vi "SM motor repeat TDC DS345 tw 2 soft.vi"(0 "SM Config":T5={"VISA Serial ref"="COM3", "Motor Config"={"DriveRatio (mm/rev)"=10.16, "PosLimit + (mm)"=200.0, "PosLimit - (mm)"=0.0, "EncoderRatio (count/rev)"=2000.0, "MotorType"=enum."SM17"}} {"Motor Config"."EncoderRatio (count/rev)" format="%.2f"; "Motor Config"."PosLimit - (mm)" format="%.3f"; "Motor Config"."PosLimit + (mm)" format="%.3f"; "Motor Config"."DriveRatio (mm/rev)" format="%.2f"}, 1 "Waiting time (s)":dbl=3.0, 2 "Sonication position (mm)":dbl, 3 "Moving times":dbl, 4 "Stop motion":bool, 5 "SM setting":T4={"Acceleration (mm/sec^2)"=1000.0, "Velocity (mm/sec)"=1.0, "Position (mm)"=0.0} {"Position (mm)" format="%.3f"; "Velocity (mm/sec)" format="%.3f"; "Acceleration (mm/sec^2)" format="%.3f"}, 6 "Lasting time (s)":dbl=5.0, 7 "Serial":i32=83858441, 9 "Moving parameters":T2={"Velocity (mm/s)"=0.5, "Abs position (mm)"=0.0, "Lasting time (s)"=25.0}, 11 "SRS DS345 GPIB address":string="0:18", 12 "Default setting (DS345)":T1={"Osc. Amp. (V)"=0.01, "Osc. Freq. (Hz)"=1000.0} {"Osc. Freq. (Hz)" min=0.001 max=250000.0 step=0.001 format="%.3f"; "Osc. Amp. (V)" min=0.0 max=0.1 step=0.001 format="%.3f"}, 13 "Cluster":T1={"Osc. Amp. (V)"=0.06, "Osc. Freq. (Hz)"=1200.0} {"Osc. Freq. (Hz)" min=0.001 max=250000.0 step=0.001 format="%.3f"; "Osc. Amp. (V)" min=0.0 max=10.0 step=0.001 format="%.3f"}, 14 "Move":bool) -> (10 "Status":T3, 15 "Position (mm)":dbl)   [LabVIEW 2015]
uses:
  magnetometers/smi/labview/CPM20Software/SmartMotor.llb/SM Config.ctl
  magnetometers/smi/labview/CPM20Software/SmartMotor.llb/SM MotorConfig.ctl
  magnetometers/smi/labview/CPM20Software/SmartMotor.llb/SM Status.ctl
  Global vab.vi
panel:
  in  "Sonication":bool
  out "Ccurrent times":dbl
  in  "Action":bool
  # "SM motor setting"
  # "TDC001 motor information"
  # "DS345 information"
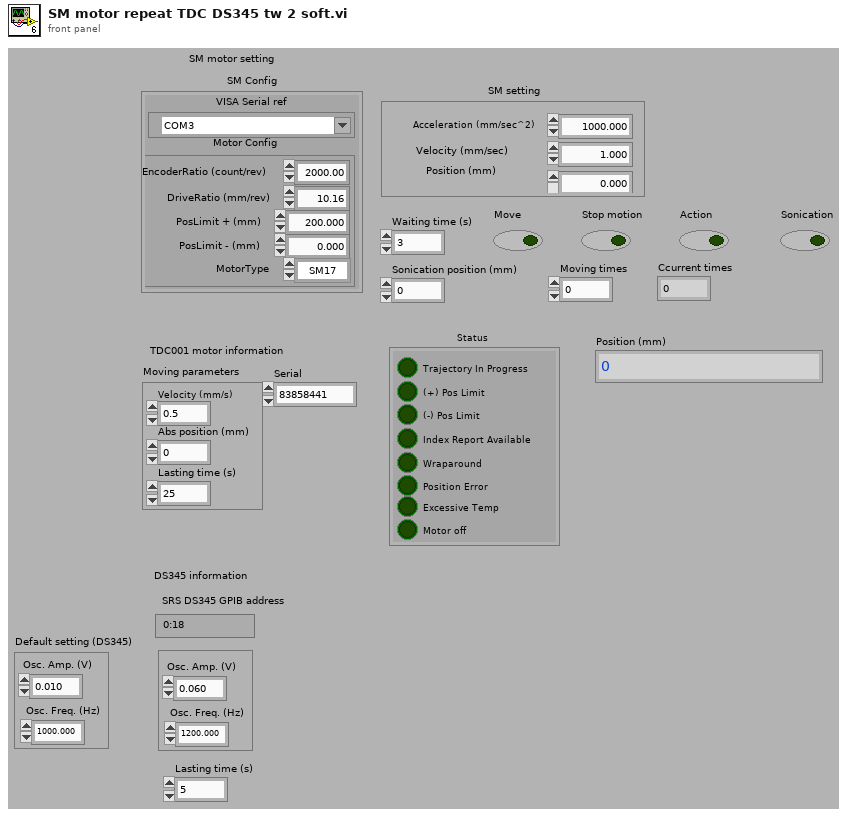
[diagram p1: front panel]
types:
  T1 = cluster{"Osc. Amp. (V)":dbl, "Osc. Freq. (Hz)":dbl}
  T2 = cluster{"Velocity (mm/s)":dbl, "Abs position (mm)":dbl, "Lasting time (s)":dbl}
  T3 = typedef "SM Status.ctl" = cluster{"Trajectory In Progress":bool, "(+) Pos Limit":bool, "(-) Pos Limit":bool, "Index Report Available":bool, "Wraparound":bool, "Position Error":bool, "Excessive Temp":bool, "Motor off":bool}
  T4 = cluster{"Acceleration (mm/sec^2)":dbl, "Velocity (mm/sec)":dbl, "Position (mm)":dbl}
  T5 = typedef "SM Config.ctl" = cluster{"VISA Serial ref":refnum<visa-resource-name>, "Motor Config":T6}
  T6 = typedef "SM MotorConfig.ctl" = cluster{"DriveRatio (mm/rev)":dbl, "PosLimit + (mm)":dbl, "PosLimit - (mm)":dbl, "EncoderRatio (count/rev)":dbl, "MotorType":enum16{"SM17", "SM23", "SM34", "SM42", "SM56"}}
  T7 = cluster{"Acceleration (mm/sec^2)":dbl, "Velocity (mm/sec)":dbl, "Sonication position (mm)":dbl}
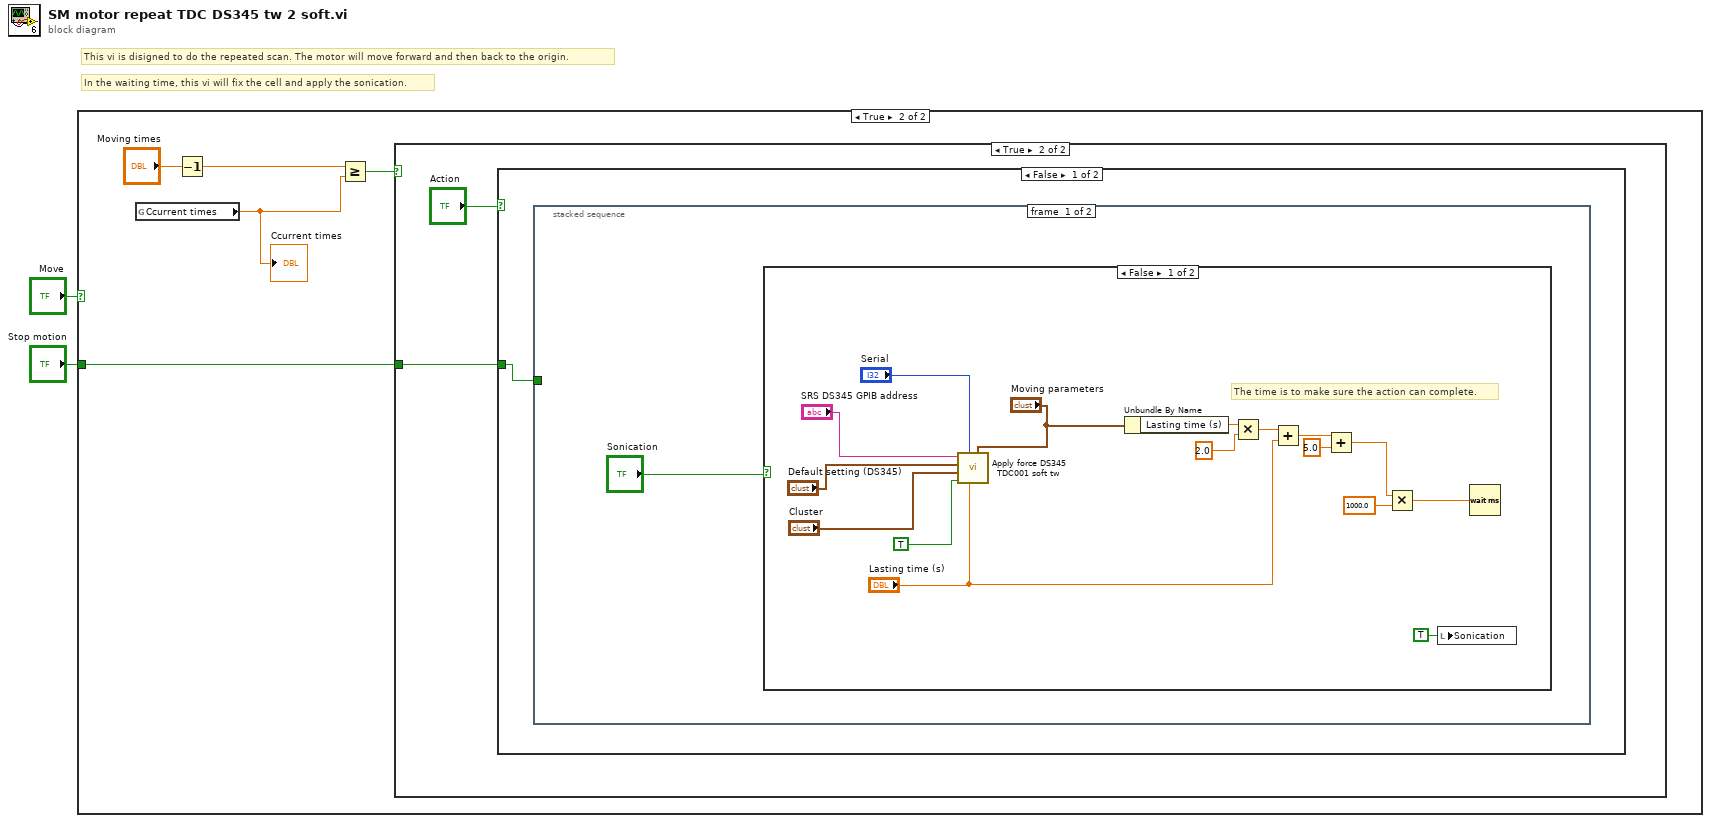
[diagram p0: block diagram]
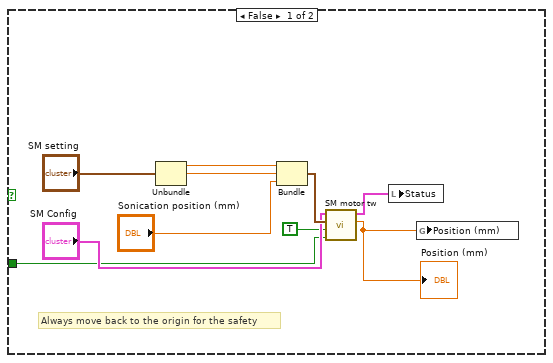
[diagram p2: hidden frame]
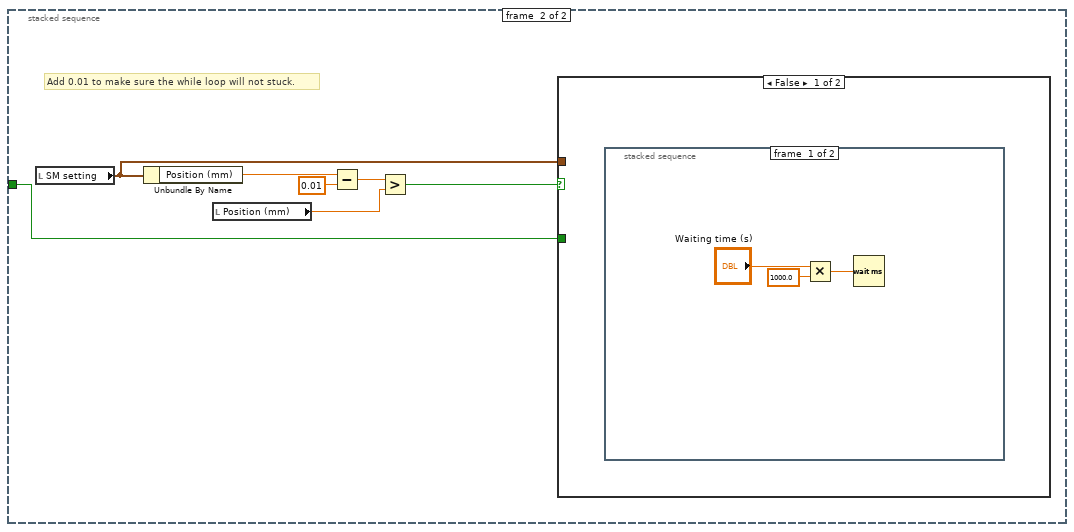
[diagram p5: hidden frame]
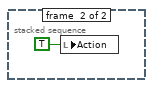
[diagram p6: hidden frame]
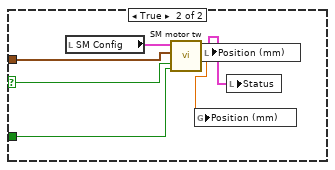
[diagram p7: hidden frame]
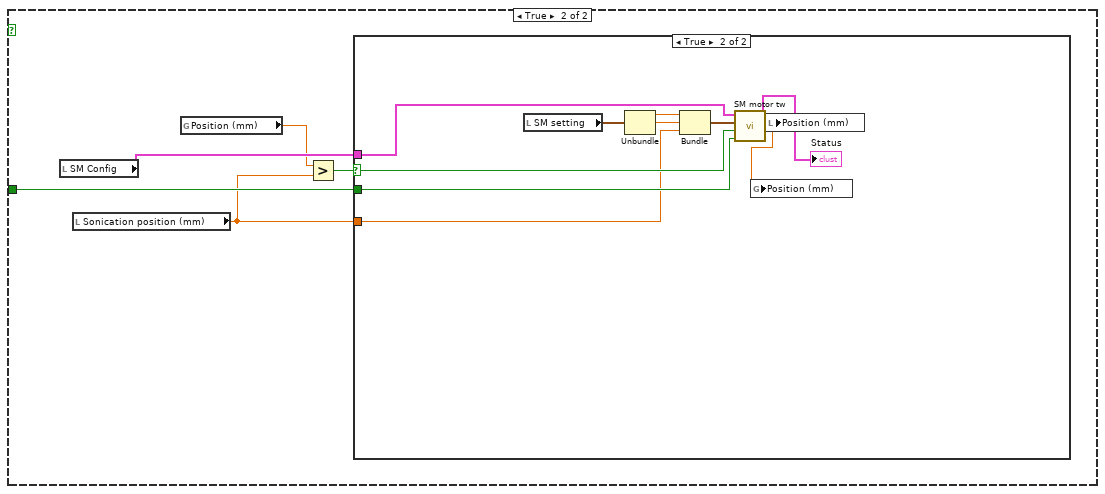
[diagram p8: hidden frame]
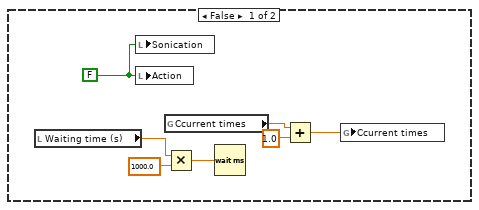
[diagram p9: hidden frame]
diagram:
  # "In the waiting time, this vi will fix the cell and apply the sonication."
  # "This vi is disigned to do the repeated scan. The motor will move forward and then back to the origin."
  n1 = case shown="True" "Move" {
    tunnel: "Stop motion" -> [w6 w15]
    frame False {
      # "Always move back to the origin for the safety"
      n2 = Unbundle("SM setting") -> ("Acceleration (mm/sec^2)"=w12:dbl, "Velocity (mm/sec)"=w11:dbl)  [unwired: 1 out]
      n3 = Bundle("Acceleration (mm/sec^2)"=w12, "Velocity (mm/sec)"=w11, "Sonication position (mm)"="Sonication position (mm)") -> (w10:T7)  [unwired: 1 out]
      n4 = call "SM motor tw.vi"("SM Config"="SM Config", "SM setting"=w10, "Move"=TRUE, "Stop motion"=w6) -> ("Status"=w4:T3, "Position (mm)"=w5:dbl)  [unwired: 5 out]
      "Position (mm)" <- w5
      n5 = local write "Status"(w4) -> ()
      n6 = global write "Global vab.vi" "Position (mm)"(w5) -> ()
    }
    frame True {
      n7 = global read "Global vab.vi" "Ccurrent times"() -> (w13:dbl)
      "Ccurrent times" <- w13
      n8 = Decrement(x="Moving times") -> (x-1=w14:dbl)
      n9 = Greater Or Equal?(x=w14, y=w13) -> (x >= y?=w16:bool)
      n10 = case shown="True" w16 {
        tunnel: w15 -> [_ w19]
        frame False {
        }
        frame True {
          n11 = case shown="False" "Action" {
            tunnel: w19 -> [w20 w57]
            frame False {
              n12 = stacked-sequence {
                tunnel: w20 -> [_ w39]
                frame #0 {
                  n13 = case shown="False" "Sonication" {
                    frame False {
                      # "The time is to make sure the action can complete."
                      n14 = call "Apply force DS345 TDC001 soft tw.vi"("Moving parameters"="Moving parameters", "Lasting time (s)"="Lasting time (s)", "TDC001 motor Serial"="Serial", "Apply force"=TRUE, "Cluster"="Cluster", "Default setting (DS345)"="Default setting (DS345)", "SRS DS345 GPIB address"="SRS DS345 GPIB address") -> ()  [unwired: 4 in]
                      n15 = Unbundle By Name("Moving parameters") -> ("Lasting time (s)"=w28:dbl)
                      n16 = Multiply(x=w28, y=2.0) -> (x*y=w26:dbl)
                      n17 = Add(x=w26, y="Lasting time (s)") -> (x+y=w24:dbl)
                      n18 = Add(x=w24, y=5.0) -> (x+y=w22:dbl)
                      n19 = Multiply(x=w22, y=1000.0) -> (x*y=w32:dbl)
                      n20 = local write "Sonication"(TRUE ("Sonication")) -> ()
                      n21 = Wait (ms)(milliseconds to wait=w32) -> ()  [unwired: 1 out]
                    }
                    frame True {
                    }
                  }
                }
                frame #1 {
                  # "Add 0.01 to make sure the while loop will not stuck."
                  n22 = local read "SM setting"() -> (w40:T4)
                  n23 = Unbundle By Name(w40) -> ("Position (mm)"=w43:dbl)
                  n24 = local read "Position (mm)"() -> (w38:dbl)
                  n25 = Subtract(x=w43, y=0.01) -> (x-y=w42:dbl)
                  n26 = Greater?(x=w42, y=w38) -> (0:w41:bool)
                  n27 = case shown="False" w41 {
                    selector: w41 -> [_ w52]
                    tunnel: w40 -> [_ w53]
                    tunnel: w39 -> [_ w51]
                    frame False {
                      n28 = stacked-sequence {
                        frame #0 {
                          n29 = Multiply(x="Waiting time (s)", y=1000.0) -> (x*y=w47:dbl)
                          n30 = Wait (ms)(milliseconds to wait=w47) -> ()  [unwired: 1 out]
                        }
                        frame #1 {
                          n31 = local write "Action"(TRUE ("Action")) -> ()
                        }
                      }
                    }
                    frame True {
                      n32 = local read "SM Config"() -> (w54:T5)
                      n33 = call "SM motor tw.vi"("SM Config"=w54, "SM setting"=w53, "Move"=w52, "Stop motion"=w51) -> ("Status"=w49:T3, "Position (mm)"=w50:dbl)  [unwired: 5 out]
                      n34 = global write "Global vab.vi" "Position (mm)"(w50) -> ()
                      n35 = local write "Position (mm)"(w50) -> ()
                      n36 = local write "Status"(w49) -> ()
                    }
                  }
                }
              }
            }
            frame True {
              n37 = local read "SM Config"() -> (w58:T5)
              n38 = local read "Sonication position (mm)"() -> (w55:dbl)
              n39 = global read "Global vab.vi" "Position (mm)"() -> (w56:dbl)
              n40 = Greater?(x=w56, y=w55) -> (0:w59:bool)
              n41 = case shown="True" w59 {
                selector: w59 -> [_ w72]
                tunnel: w58 -> [_ w71]
                tunnel: w57 -> [_ w70]
                tunnel: w55 -> [_ w67]
                frame False {
                  w60 = FALSE ("Action")
                  n42 = local read "Waiting time (s)"() -> (w61:dbl)
                  n43 = local write "Sonication"(w60) -> ()
                  n44 = local write "Action"(w60) -> ()
                  n45 = global read "Global vab.vi" "Ccurrent times"() -> (w64:dbl)
                  n46 = Multiply(x=w61, y=1000.0) -> (x*y=w62:dbl)
                  n47 = Wait (ms)(milliseconds to wait=w62) -> ()  [unwired: 1 out]
                  n48 = Add(x=w64, y=1.0) -> (x+y=w65:dbl)
                  n49 = global write "Global vab.vi" "Ccurrent times"(w65) -> ()
                }
                frame True {
                  n50 = local read "SM setting"() -> (w73:T4)
                  n51 = Unbundle(w73) -> ("Acceleration (mm/sec^2)"=w74:dbl, "Velocity (mm/sec)"=w75:dbl)  [unwired: 1 out]
                  n52 = Bundle("Acceleration (mm/sec^2)"=w74, "Velocity (mm/sec)"=w75, "Sonication position (mm)"=w67) -> (w76:T7)  [unwired: 1 out]
                  n53 = call "SM motor tw.vi"("SM Config"=w71, "SM setting"=w76, "Move"=w72, "Stop motion"=w70) -> ("Status"=→"Status":T3, "Position (mm)"=w69:dbl)  [unwired: 5 out]
                  n54 = global write "Global vab.vi" "Position (mm)"(w69) -> ()
                  n55 = local write "Position (mm)"(w69) -> ()
                }
              }
            }
          }
        }
      }
    }
  }
